vi "Start Heartbeats.vi"(8 "error in":errorcluster, 11 "CANopen in":refnum<class "CANopen.lvclass">) -> (0 "error out":errorcluster, 3 "CANopen out":refnum<class "CANopen.lvclass">)   [LabVIEW 2024, in "canopen.lvlib" / "CANopen.lvclass"]
doc: "Starts the generation of heartbeat messages from a specific node or from all the nodes stored in the heartbeat table if \"Node ID\" is not specified."
uses:
  CANopen.lvclass
  CANopen.lvclass/CANopen.ctl
  Multiplexor.ctl
  CANopen Master.lvlib
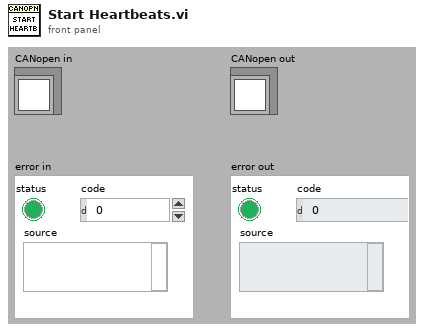
[diagram p1: front panel]
types:
  T1 = typedef "CANopen Master.lvlib/Multiplexor.ctl" = cluster{"Index":u16, "Sub-Index":u8}
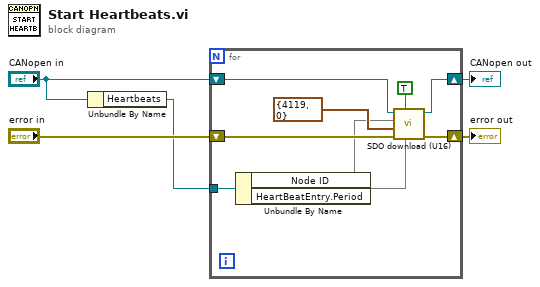
[diagram p0: block diagram]
diagram:
  n1 = Unbundle By Name("CANopen in") -> ("Heartbeats"=w1:refnum<data-value>)
  n2 = for {
    tunnel: w1 -> [w11]
    shift-right: [w13] -> w3
    shift-left: "error in" -> [w14]
    shift-right: [w10] -> w2
    shift-left: "CANopen in" -> [w12]
    n3 = Unbundle By Name(w11) -> ("Node ID"=w7, "HeartBeatEntry.Period"=w8)
    n4 = call "SDO download (U16).vi"("Value"=w8, "Wait?"=TRUE, "error in"=w14, "Multiplexor"=T1 {"Index"=4119, "Sub-Index"=0}, "Node ID"=w7, "CANopen in"=w12) -> ("error out"=w13:errorcluster, "CANopen out"=w10:refnum<class "CANopen.lvclass">)  [unwired: 4 in]
  }
  "CANopen out" <- w2
  "error out" <- w3
